vi "Example Callback.vi"() -> ()   [LabVIEW 2013]
uses:
  C:/tf/play/labview/Tinkerforge.dll
  Tinkerforge.dll
panel:
  in  "stop":bool
  out "CO2 concentration (ppm)":i32
  in  "uid":string="amb"
  in  "port":i32=4223
  in  "host":string="localhost"
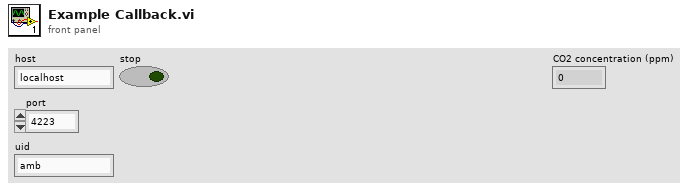
[diagram p1: front panel]
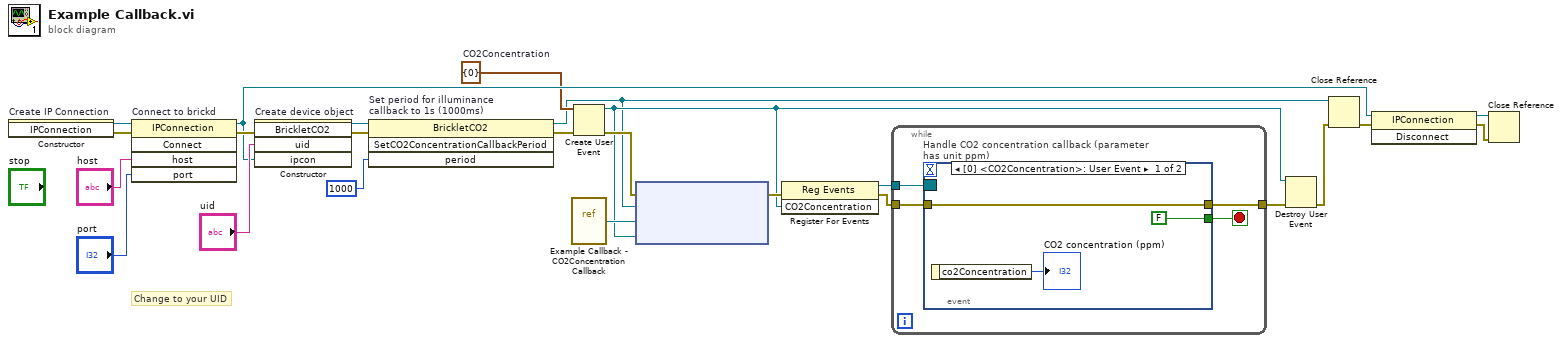
[diagram p0: block diagram]
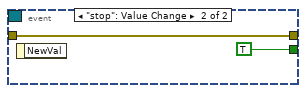
[diagram p2: hidden frame]
diagram:
  w7 = cluster{"co2Concentration":i32} {"co2Concentration"=0}  # CO2Concentration
  # "Change to your UID"
  n1 = constructor on="Create IP Connection" class="IPConnection"() -> (reference out=w24:refnum<k24>, error out=w1:errorcluster)  [unwired: 3 in, 1 out]
  n2 = invoke on="Connect to brickd" class="IPConnection" method="Connect"(reference=w24, error in=w1, "host"="host", "port"="port") -> (reference out=w17:refnum<k24>, error out=w20:errorcluster)  [unwired: 1 in, 3 out]
  n3 = constructor on="Create device object" class="BrickletCO2"(error in=w20, "uid"="uid", "ipcon"=w17) -> (reference out=w4:refnum<k24>, error out=w6:errorcluster)  [unwired: 2 in, 3 out]
  n4 = invoke on="Set period for illuminance\ncallback to 1s (1000ms)" class="BrickletCO2" method="SetCO2ConcentrationCallbackPeriod"(reference=w4, error in=w6, "period"=i64 1000) -> (reference out=w3:refnum<k24>, error out=w5:errorcluster)  [unwired: 1 in, 2 out]
  n5 = vi-ref "Example Callback - CO2Concentration Callback.vi"() -> ("vi reference"=w13:refnum<vi>)
  n6 = Create User Event(user event datatype=w7, error in=w5) -> (user event=w9:refnum<user-event>, error out=w15:errorcluster)
  n7 = node ("Register Event Callback")(w15, w3, w13, w9) -> (w14:errorcluster)  [unwired: 1 in, 1 out]
  n8 = register-events(error in=w14, w9) -> (reference out=w12:refnum<event-registration>, error out=w10:errorcluster)  [unwired: 1 in]
  n9 = while {
    tunnel: w12 -> [w28]
    tunnel: [w27] -> w11
    tunnel: w10 -> [w26]
    stop <- w25 stop-if-true
    n10 = event "Handle CO2 concentration callback (parameter has unit ppm)" shown="[0] <CO2Concentration>: User Event" {
      selector: w28 -> [_ _]
      dyn-events: _ -> [_ _]
      timeout: _ -> [_ _]
      tunnel: [w31 w32] -> w27
      tunnel: w26 -> [w31 w32]
      tunnel: [FALSE TRUE] -> w25
      event User Event {
        n11 = event-data() -> ("co2Concentration"=→"CO2 concentration (ppm)":i32)  [unwired: 1 in]
      }
      event "stop": Value Change {
        n12 = event-data() -> ()  [unwired: 1 in, 1 out]
      }
    }
  }
  n13 = Destroy User Event(user event=w9, error in=w11) -> (error out=w8:errorcluster)
  n14 = Close Reference(reference=w3, error in (no error)=w8) -> (error out=w19:errorcluster)
  n15 = invoke class="IPConnection" method="Disconnect"(reference=w17, error in=w19) -> (reference out=w16:refnum<k24>, error out=w18:errorcluster)  [unwired: 1 in, 1 out]
  n16 = Close Reference(reference=w16, error in (no error)=w18) -> ()  [unwired: 1 out]
